vi "CalculateFluence.vi"(9 "Period (s)":dbl, 10 "Flux (ions/s * cm^2)":dbl, 11 "Fluence In (ions/cm^2)":dbl) -> (3 "Fluence Out (ions/cm^2)":dbl)   [LabVIEW 2012]
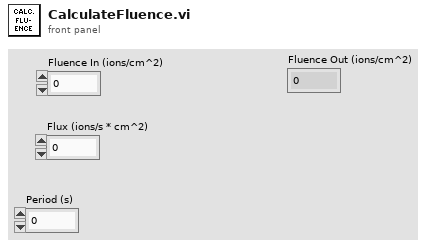
[diagram p1: front panel]
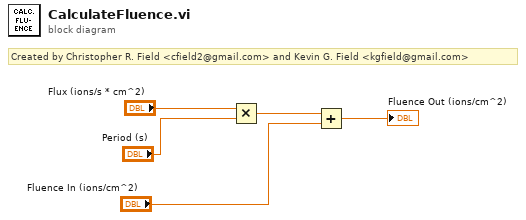
[diagram p0: block diagram]
diagram:
  # "Created by Christopher R. Field <cfield2@gmail.com> and Kevin G. Field <kgfield@gmail.com>"
  n1 = Multiply(x="Flux (ions/s * cm^2)", y="Period (s)") -> (x*y=w3:dbl)
  n2 = Add(x=w3, y="Fluence In (ions/cm^2)") -> (x+y=→"Fluence Out (ions/cm^2)":dbl)
